vi "Run Step.vi"(8 "error in (no error)":errorcluster, 9 "result allocation":T1, 10 "parameters":T1, 11 "Parallel Step in":refnum<class "Parallel Step.lvclass">) -> (0 "error out":errorcluster, 1 "results":T1, 2 "parameter allocation":T1, 3 "Parallel Step out":refnum<class "Parallel Step.lvclass">)   [LabVIEW 2015, in "Parallel Step.lvclass"]
uses:
  Parallel Step.lvclass
  <vilib>/NI/Tag Bus/table/data table.ctl
  Step/StepState.ctl
  Step/Step State Enum.ctl
  Step/Step Flow Control.ctl
  Step/Step.lvclass
  <vilib>/NI/Tag Bus/table/data table.lvlib
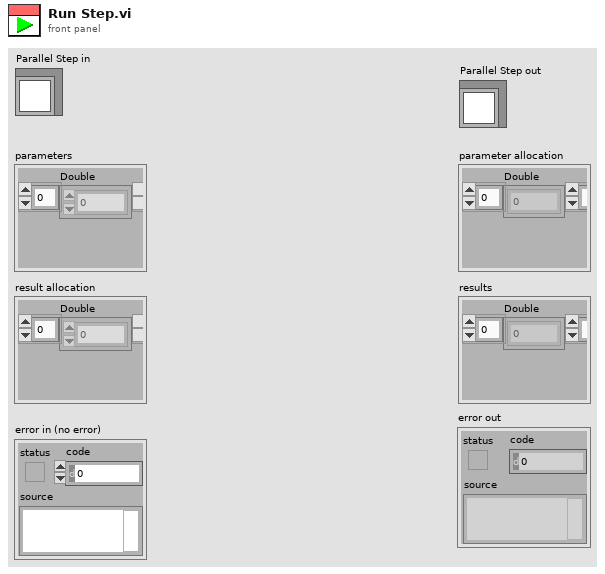
[diagram p1: front panel]
types:
  T1 = typedef "tag bus.lvlib/data table.lvlib/data table.ctl" = cluster{"Double":dbl[], "Single":sgl[], "I64":i64[], "I32":i32[], "I16":i16[], "I8":i8[], "U64":u64[], "U32":u32[], "U16":u16[], "U8":u8[], "Boolean":bool[], "String":string[], "Array of Double":cluster{"DBL Array":dbl[]}[], "Array of Single":cluster{"SGL Array":sgl[]}[], "Array of I64":cluster{"I64 Array":i64[]}[], "Array of I32":cluster{"I32 Array":i32[]}[], "Array of I16":cluster{"I16 Array":i16[]}[], "Array of I8":cluster{"I8 Array":i8[]}[], "Array of U64":cluster{"U64 Array":u64[]}[], "Array of U32":cluster{"U32 Array":u32[]}[], "Array of U16":cluster{"U16 Array":u16[]}[], "Array of U8":cluster{"U8 Array":u8[]}[], "Array of Boolean":cluster{"Boolean Array":bool[]}[], "Array of String":cluster{"String Array":string[]}[]}
  T2 = typedef "Step.lvclass/StepState.ctl" = cluster{"Step State":T3, "Flow Control":T4, "Index":i32}
  T3 = typedef "Step.lvclass/Step State Enum.ctl" = enum16{"Start", "Skipped", "Completed", "Running", "Aborted"}
  T4 = typedef "Step.lvclass/Step Flow Control.ctl" = enum16{"Next Step", "Jump"}
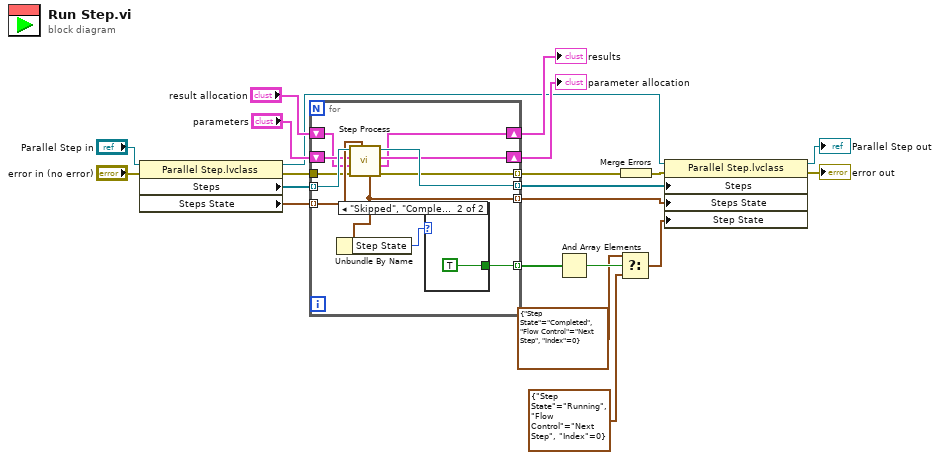
[diagram p0: block diagram]
diagram:
  n1 = property class="Parallel Step.lvclass"(reference="Parallel Step in", error in="error in (no error)") -> (reference out=w11:refnum<class "Parallel Step.lvclass">, error out=w7:errorcluster, "Steps"=w20:refnum<class "Step.lvclass">[], "Steps State"=w19:T2[])
  n2 = for {
    tunnel: w20 -> [w33] mode=indexing
    tunnel: w19 -> [w31] mode=indexing
    tunnel: [w32] -> w18 mode=indexing
    tunnel: [w23] -> w17 mode=indexing
    tunnel: [w26] -> w12 mode=indexing
    tunnel: w7 -> [w25]
    shift-right: [w28] -> w14
    shift-left: "parameters" -> [w30]
    shift-right: [w27] -> w13
    shift-left: "result allocation" -> [w29]
    tunnel: [w24] -> w5 mode=indexing
    n3 = call-dynamic "Step Process.vi"("Step State in"=w31, "error in (no error)"=w25, "result allocation"=w29, "parameters"=w30, "Step in"=w33) -> ("error out"=w26:errorcluster, "results"=w27:T1, "parameter allocation"=w28:T1, "Step out"=w32:refnum<class "Step.lvclass">, "Step State out"=w23:T2)  [unwired: 2 in]
    n4 = Unbundle By Name(w23) -> ("Step State"=w22:T3)
    n5 = case shown="\"Skipped\", \"Completed\"" w22 {
      tunnel: [_ TRUE] -> w24
      frame "Start", Default {
      }
      frame "Skipped", "Completed" {
      }
    }
  }
  "results" <- w13
  "parameter allocation" <- w14
  n6 = And Array Elements(Boolean array=w5) -> (logical AND=w4:bool)
  n7 = Select(t=T2 {"Step State"=enum."Completed", "Flow Control"=enum."Next Step", "Index"=0} ("Step State"), s=w4, f=T2 {"Step State"=enum."Running", "Flow Control"=enum."Next Step", "Index"=0} ("Step State")) -> (s? t:f=w2:T2)
  n8 = Merge Errors(w12) -> (w9:errorcluster)
  n9 = property class="Parallel Step.lvclass"(reference=w11, error in=w9, "Steps"=w18, "Steps State"=w17, "Step State"=w2) -> (reference out=→"Parallel Step out":refnum<class "Parallel Step.lvclass">, error out=→"error out":errorcluster)
